vi "followUpDevice.vi"(8 "error in (no error)":errorcluster, 9 "S/N":string, 10 "Device Type":T1=enum."k4b2", 11 "reference in":refnum<class "Project Panels.lvclass">) -> (0 "error out":errorcluster, 3 "reference out":refnum<class "Project Panels.lvclass">)   [LabVIEW 2016, in "Project Panels.lvclass"]
uses:
  Project Panels.lvclass
  SYS/Devices Controller_llb/deviceType.ctl
  SYS/Devices Controller_llb/Devices Controller.lvclass
  SYS/File Controller_llb/File Controller.lvclass
  SYS/Notification Controller_class/Notification Controller.lvclass
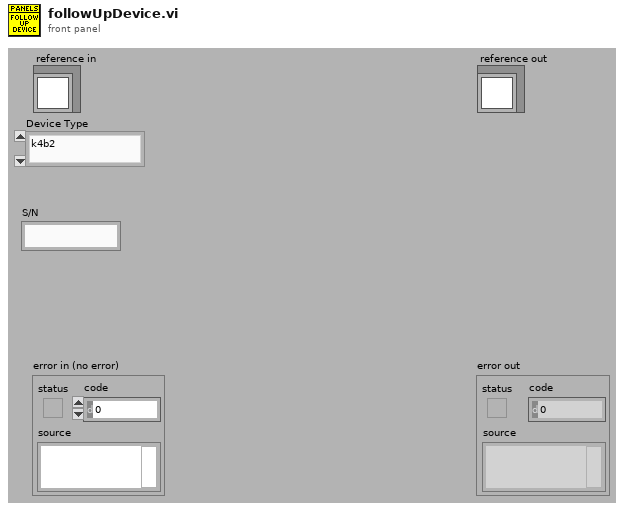
[diagram p1: front panel]
types:
  T1 = typedef "Devices Controller.lvclass/deviceType.ctl" = enum16{"k5", "k4b2", "fitmate", "cpet", "rmr", "bodyBoxPft", "bp", "pp"}
  T2 = typedef "Project Panels.lvclass/ObjectAttributesRef.ctl" = refnum<data-value>
  T3 = typedef "Project Panels.lvclass/ObjectAttributes.ctl" = cluster{"MyAttribute":dbl, "device_controller_ref":refnum<class "Devices Controller.lvclass">, "file_controller_ref":refnum<class "File Controller.lvclass">, "item_controller_ref":refnum<class "Items Controller.lvclass">, "item_tables":cluster{"checkIN":string[][], "checkOUT":string[][], "storage":string[][]}, "quickbook_table":cluster{"notes":string[][]}, "notification_controller_ref":refnum<class "Notification Controller.lvclass">, "partstracking_controller_ref":refnum<class "PartsTracking Controller.lvclass">, "product_tables":cluster{"k4b2":string[][], "fitmate":string[][], "RMR":string[][], "CPET":string[][], "BP":string[][], "PP":string[][], "k5":string[][], "bb-pft":string[][]}, "rowsColour":u32[], "low_resolution?":bool, "run_python?":bool}
  T4 = cluster{"deviceType":T1, "S/N":string, "SW":string, "Description":string, "Account":string, "System's Location":string, "End User":string, "Email":string, "City":string, "LastChange":string, "Service By":string, "Exp Date":string, "FollowUp Sent":string, "FollowUp Accepted":string, "Note":string}
  T5 = cluster{"filePaths":path[], "outlookTemplatePaths":path[], "attachmentTemplatePaths":path[]}
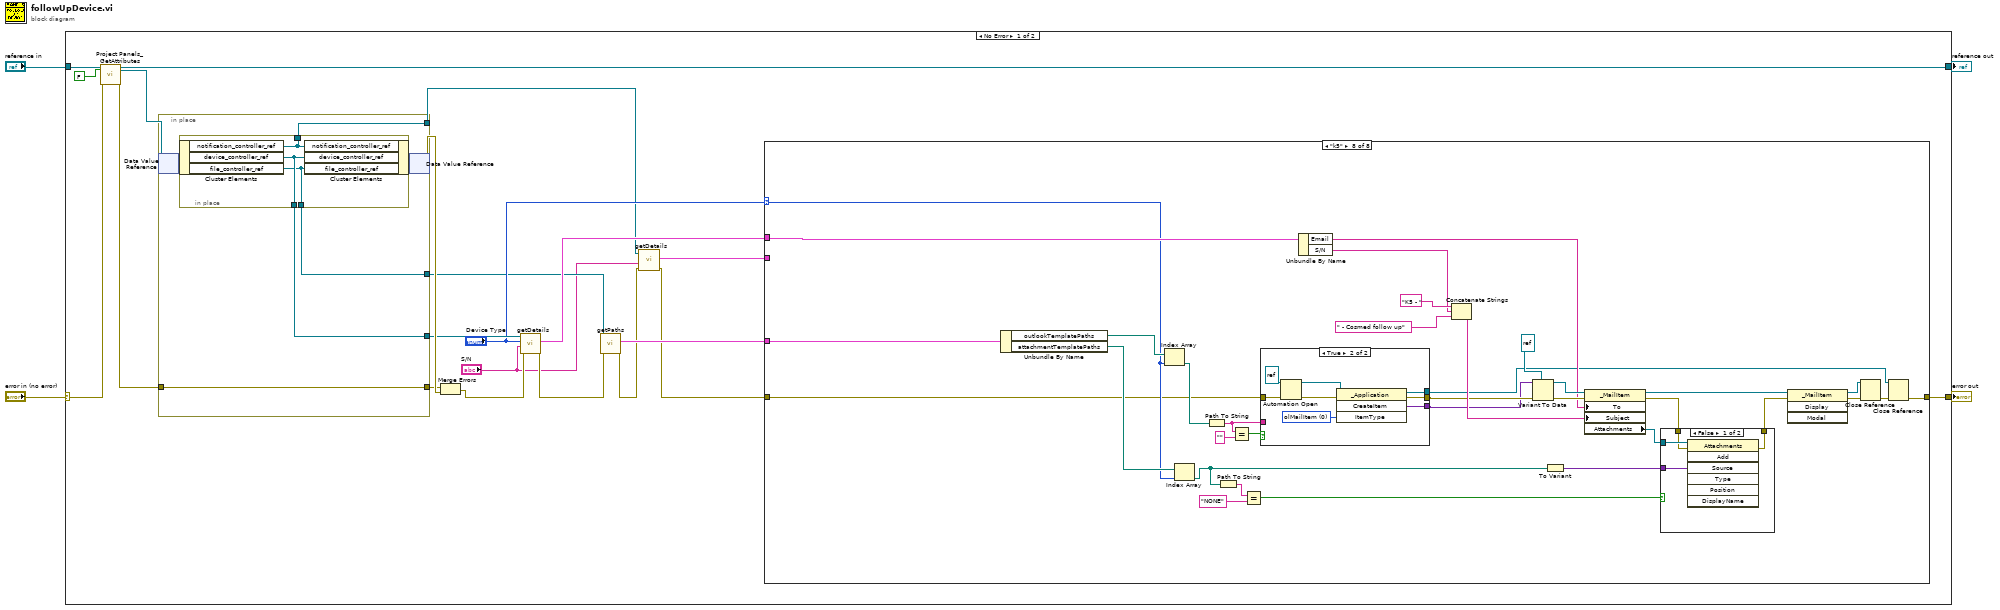
[diagram p0: block diagram]
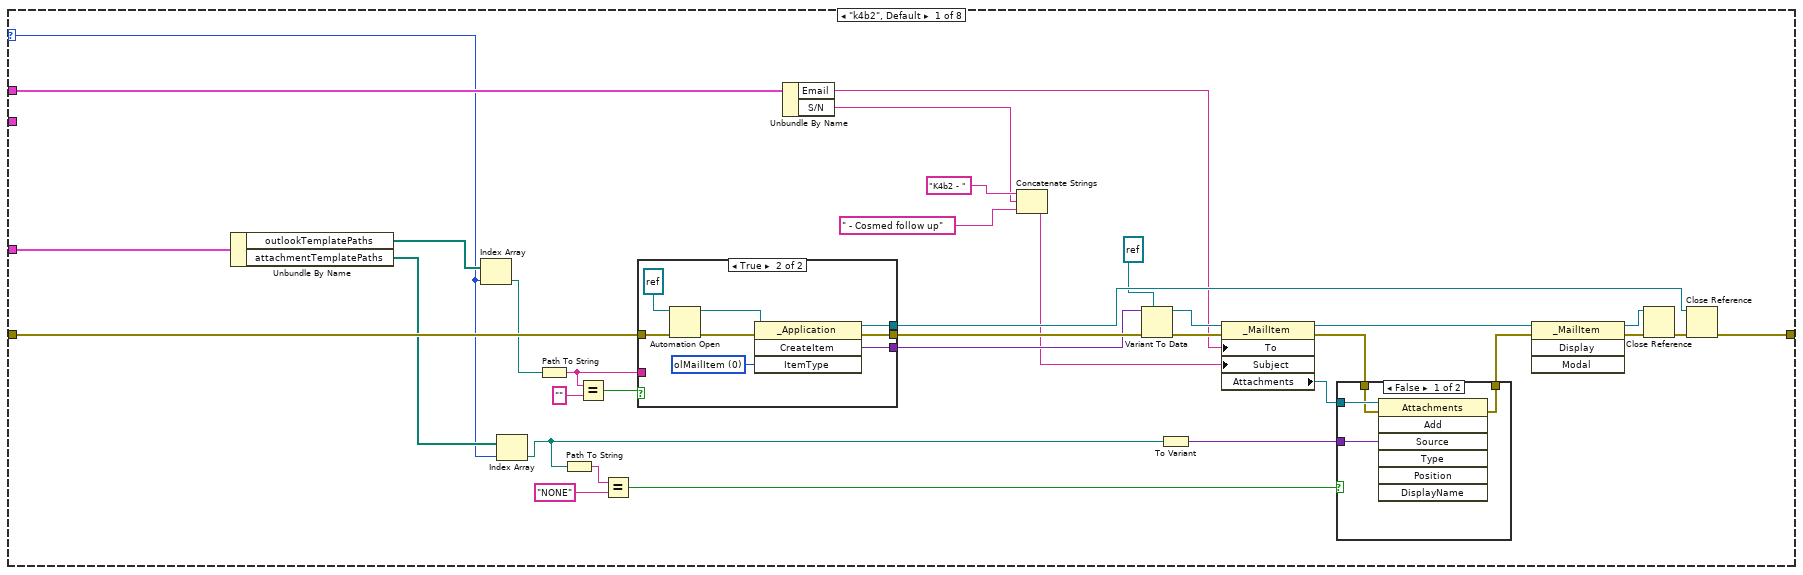
[diagram p2: hidden frame]
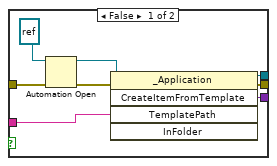
[diagram p3: hidden frame]
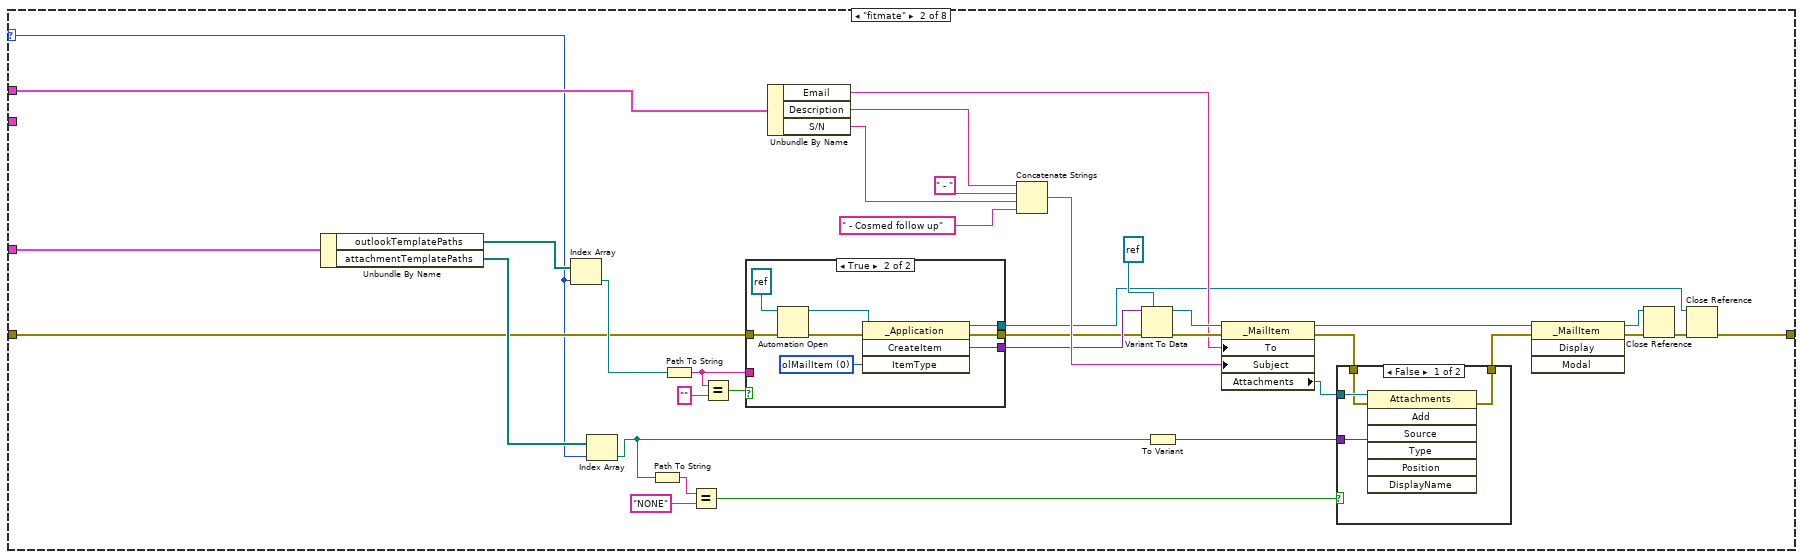
[diagram p5: hidden frame]
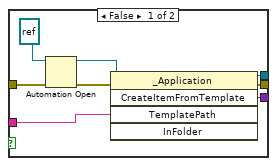
[diagram p6: hidden frame]
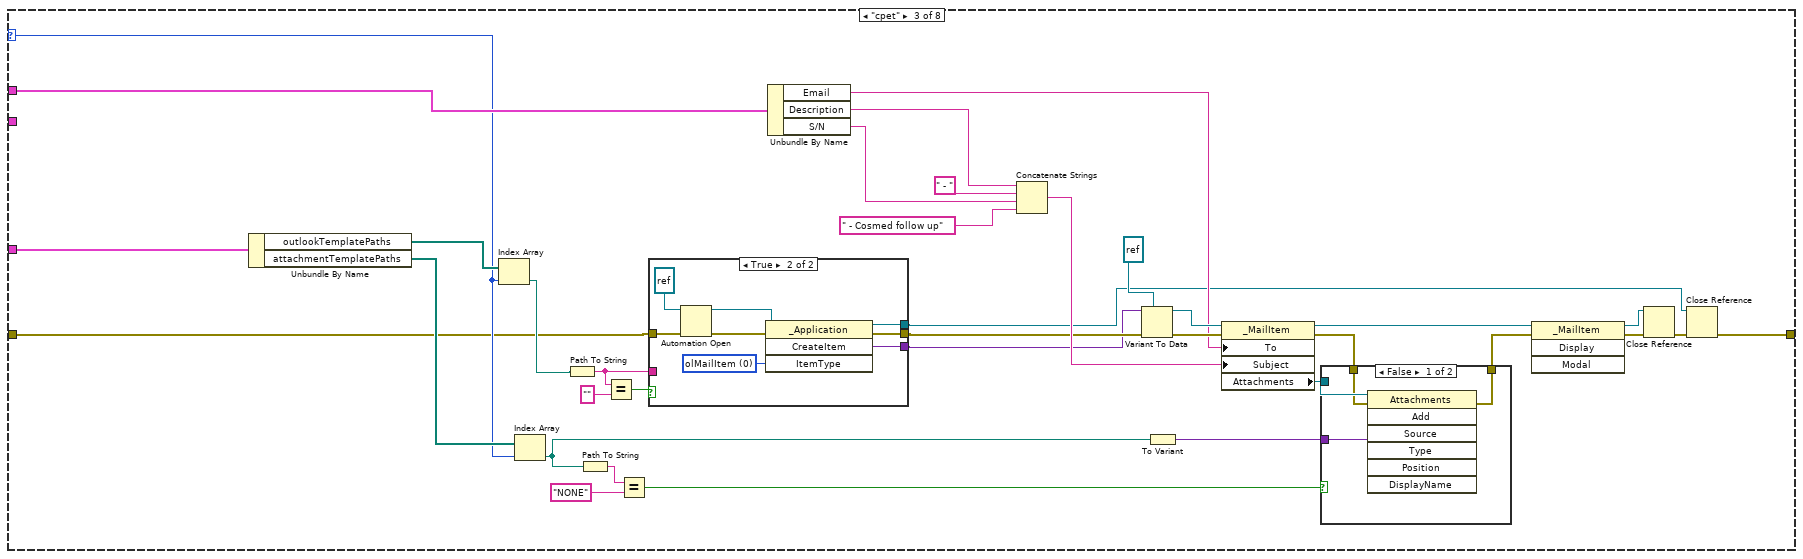
[diagram p8: hidden frame]
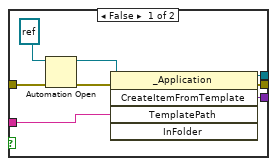
[diagram p9: hidden frame]
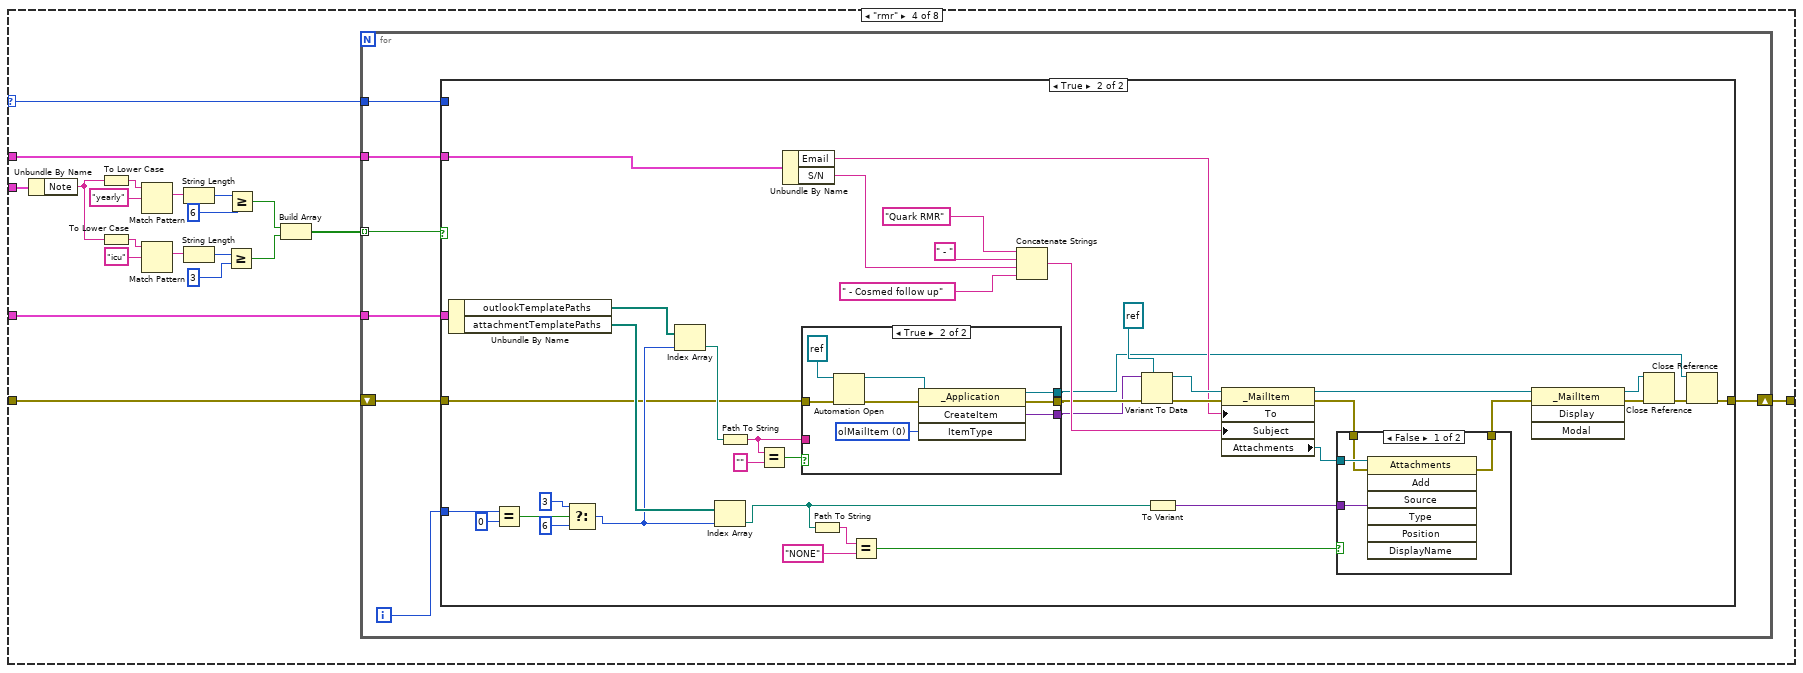
[diagram p11: hidden frame]
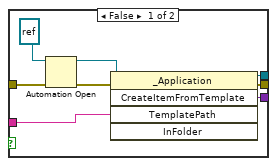
[diagram p13: hidden frame]
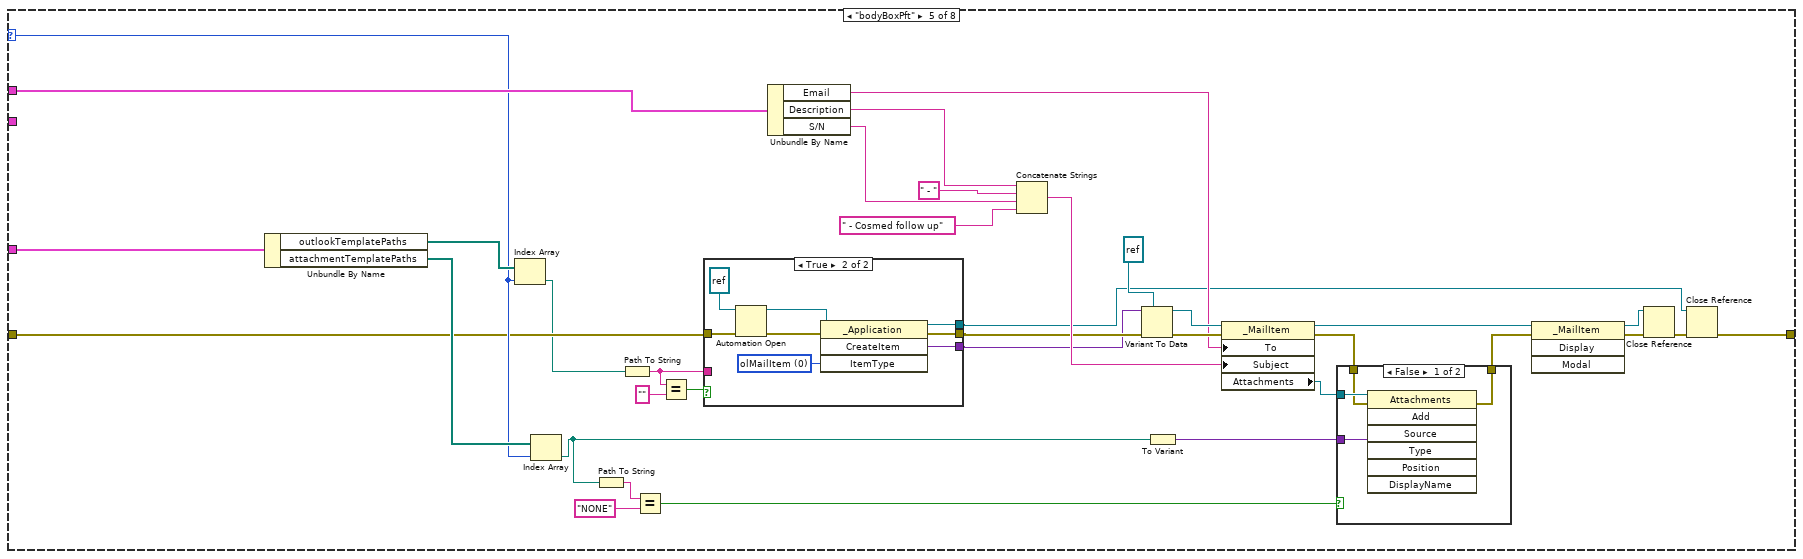
[diagram p15: hidden frame]
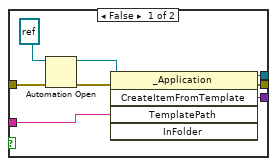
[diagram p16: hidden frame]
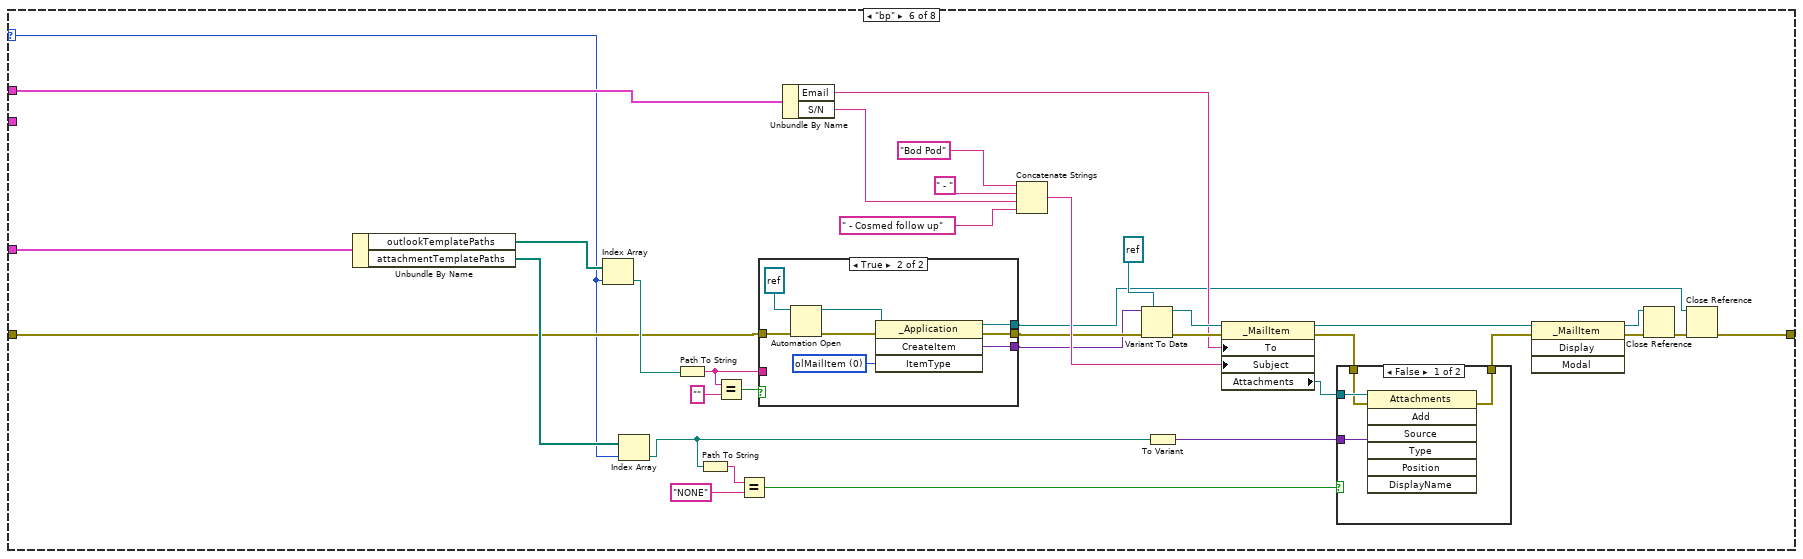
[diagram p18: hidden frame]
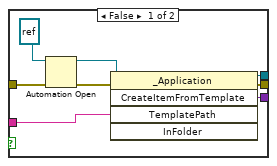
[diagram p19: hidden frame]
diagram:
  n1 = case shown="No Error" "error in (no error)" {
    selector: "error in (no error)" -> [w21 w514]
    tunnel: [w17 w514] -> w3
    tunnel: [w19 w513] -> w1
    tunnel: "reference in" -> [w23 w513]
    frame No Error {
      n2 = call "Project Panels_GetAttributes.vi"("reference in"=w23, "return data? (T)"=FALSE, "error in (no error)"=w21) -> ("reference out"=w19:refnum<class "Project Panels.lvclass">, "attributes ref"=w18:T2, "error out"=w20:errorcluster)  [unwired: 13 in, 1 out]
      n3 = in-place {
        in-place-border: w20 -> [w507]
        in-place-border: [w507] -> w24
        in-place-border: [w506] -> w15
        in-place-border: [w505] -> w12
        in-place-border: [w504] -> w5
        n4 = in-place-dvr #1(w18) -> (w508:T3)  [unwired: 1 out]
        n5 = in-place {
          in-place-border: [w512] -> w506
          in-place-border: [w511] -> w505
          in-place-border: [w510] -> w504
          n6 = in-place-cluster #2(w508) -> ("notification_controller_ref"=w510:refnum<class "Notification Controller.lvclass">, "device_controller_ref"=w512:refnum<class "Devices Controller.lvclass">, "file_controller_ref"=w511:refnum<class "File Controller.lvclass">)
          n7 = in-place-cluster #2("notification_controller_ref"=w510, "device_controller_ref"=w512, "file_controller_ref"=w511) -> (w509:T3)
        }
        n8 = in-place-dvr #1(w509) -> (w25:errorcluster)  [unwired: 1 out]
      }
      n9 = Merge Errors(w24, w25) -> (w16:errorcluster)
      n10 = call "getDetails.vi"("error in (no error)"=w16, "S/N"="S/N", "Device Type"="Device Type", "reference in"=w15) -> ("error out"=w11:errorcluster, "details"=w13:T4)  [unwired: 5 in, 1 out]
      n11 = call "getPaths.vi"("error in (no error)"=w11, "reference in"=w12) -> ("error out"=w8:errorcluster, "paths"=w10:T5)  [unwired: 7 in, 1 out]
      n12 = call "getDetails.vi"("error in (no error)"=w8, "S/N"="S/N", "reference in"=w5) -> ("error out"=w7:errorcluster, "details"=w9:T4)  [unwired: 6 in, 1 out]
      n13 = case shown="\"k5\"" "Device Type" {
        selector: "Device Type" -> [w29 w81 w145 w209 w291 w338 w402 w457]
        tunnel: [w49 w108 w164 w212 w309 w365 w403 w458] -> w17
        tunnel: w7 -> [w48 w85 w140 w211 w287 w342 w397 w452]
        tunnel: w13 -> [w47 w107 w163 w207 w308 w364 w404 w459]
        tunnel: w10 -> [w37 w94 w150 w210 w296 w352 w405 w460]
        tunnel: w9 -> [_ _ _ w208 _ _ _ _]
        frame "k4b2", Default {
          n14 = Unbundle By Name(w37) -> ("outlookTemplatePaths"=w36:path[], "attachmentTemplatePaths"=w35:path[])
          n15 = Index Array(array=w36, index=w29) -> (element=w34:path)
          n16 = Index Array(array=w35, index=w29) -> (element=w33:path)
          n17 = Path To String(path=w34) -> (string=w28:string)
          n18 = Path To String(path=w33) -> (string=w32:string)
          n19 = Equal?(x=w28, y="") -> (x = y?=w26:bool)
          n20 = Equal?(x=w32, y="NONE") -> (x = y?=w30:bool)
          n21 = case shown="True" w26 {
            tunnel: [w66 w69] -> w56
            tunnel: [w65 w70] -> w55
            tunnel: [w63 w71] -> w54
            tunnel: w48 -> [w61 w72]
            tunnel: w28 -> [w60 _]
            frame False {
              n22 = Automation Open(error in (no error)=w61, Automation Refnum=refnum<k7> refnum ("Outlook._Application")) -> (Automation Refnum=w67:refnum<k7>, error out=w62:errorcluster)  [unwired: 2 in]
              n23 = invoke class="_Application" method="CreateItemFromTemplate"(reference=w67, error in=w62, "TemplatePath"=w60) -> (reference out=w66:refnum<k7>, error out=w65:errorcluster, "CreateItemFromTemplate"=w63:variant)  [unwired: 2 in, 2 out]
            }
            frame True {
              w68 = 0 items=["olMailItem"=0, "olAppointmentItem"=1, "olContactItem"=2, "olTaskItem"=3, "olJournalItem"=4, "olNoteItem"=5, "olPostItem"=6, "olDistributionListItem"=7, "olMobileItemSMS"=11, "olMobileItemMMS"=12] ("ItemType")
              n24 = Automation Open(error in (no error)=w72, Automation Refnum=refnum<k7> refnum ("Outlook._Application")) -> (Automation Refnum=w75:refnum<k7>, error out=w74:errorcluster)  [unwired: 2 in]
              n25 = invoke class="_Application" method="CreateItem"(reference=w75, error in=w74, "ItemType"=w68) -> (reference out=w69:refnum<k7>, error out=w70:errorcluster, "CreateItem"=w71:variant)  [unwired: 1 in, 1 out]
            }
          }
          n26 = Unbundle By Name(w47) -> ("Email"=w46:string, "S/N"=w44:string)
          n27 = Concatenate Strings("K4b2 - " ("string"), w44, " - Cosmed follow up" ("string")) -> (w42:string)
          n28 = Variant To Data(error in=w55, type=refnum<k7> refnum ("Outlook._MailItem"), Variant=w54) -> (data=w57:refnum<k7>, error out=w50:errorcluster)
          n29 = To Variant(anything=w33) -> (Variant=w38:variant)
          n30 = property class="_MailItem"(reference=w57, error in=w50, "To"=w46, "Subject"=w42) -> (reference out=w58:refnum<k7>, error out=w40:errorcluster, "Attachments"=w41:refnum<k7>)
          n31 = case shown="False" w30 {
            tunnel: w41 -> [w79 _]
            tunnel: w40 -> [w78 w80]
            tunnel: [w77 w80] -> w39
            tunnel: w38 -> [w76 _]
            frame False {
              n32 = invoke class="Attachments" method="Add"(reference=w79, error in=w78, "Source"=w76) -> (error out=w77:errorcluster)  [unwired: 4 in, 6 out]
            }
            frame True {
            }
          }
          n33 = invoke class="_MailItem" method="Display"(reference=w58, error in=w39) -> (reference out=w52:refnum<k7>, error out=w51:errorcluster)  [unwired: 2 in, 2 out]
          n34 = Close Reference(reference=w52, error in (no error)=w51) -> (error out=w59:errorcluster)
          n35 = Close Reference(reference=w56, error in (no error)=w59) -> (error out=w49:errorcluster)
        }
        frame "fitmate" {
          n36 = Unbundle By Name(w94) -> ("outlookTemplatePaths"=w96:path[], "attachmentTemplatePaths"=w95:path[])
          n37 = Index Array(array=w96, index=w81) -> (element=w86:path)
          n38 = Index Array(array=w95, index=w81) -> (element=w91:path)
          n39 = Path To String(path=w91) -> (string=w93:string)
          n40 = Path To String(path=w86) -> (string=w89:string)
          n41 = Equal?(x=w93, y="NONE") -> (x = y?=w90:bool)
          n42 = Equal?(x=w89, y="") -> (x = y?=w87:bool)
          n43 = case shown="True" w87 {
            tunnel: [w122 w125] -> w84
            tunnel: [w121 w126] -> w82
            tunnel: [w119 w127] -> w83
            tunnel: w85 -> [w117 w128]
            tunnel: w89 -> [w116 _]
            frame False {
              n44 = Automation Open(error in (no error)=w117, Automation Refnum=refnum<k7> refnum ("Outlook._Application")) -> (Automation Refnum=w123:refnum<k7>, error out=w118:errorcluster)  [unwired: 2 in]
              n45 = invoke class="_Application" method="CreateItemFromTemplate"(reference=w123, error in=w118, "TemplatePath"=w116) -> (reference out=w122:refnum<k7>, error out=w121:errorcluster, "CreateItemFromTemplate"=w119:variant)  [unwired: 2 in, 2 out]
            }
            frame True {
              w124 = 0 items=["olMailItem"=0, "olAppointmentItem"=1, "olContactItem"=2, "olTaskItem"=3, "olJournalItem"=4, "olNoteItem"=5, "olPostItem"=6, "olDistributionListItem"=7, "olMobileItemSMS"=11, "olMobileItemMMS"=12] ("ItemType")
              n46 = Automation Open(error in (no error)=w128, Automation Refnum=refnum<k7> refnum ("Outlook._Application")) -> (Automation Refnum=w131:refnum<k7>, error out=w130:errorcluster)  [unwired: 2 in]
              n47 = invoke class="_Application" method="CreateItem"(reference=w131, error in=w130, "ItemType"=w124) -> (reference out=w125:refnum<k7>, error out=w126:errorcluster, "CreateItem"=w127:variant)  [unwired: 1 in, 1 out]
            }
          }
          n48 = Unbundle By Name(w107) -> ("Email"=w106:string, "Description"=w103:string, "S/N"=w101:string)
          n49 = Concatenate Strings(w103, " - " ("string"), w101, " - Cosmed follow up" ("string")) -> (w104:string)
          n50 = Variant To Data(error in=w82, type=refnum<k7> refnum ("Outlook._MailItem"), Variant=w83) -> (data=w113:refnum<k7>, error out=w109:errorcluster)
          n51 = To Variant(anything=w91) -> (Variant=w97:variant)
          n52 = property class="_MailItem"(reference=w113, error in=w109, "To"=w106, "Subject"=w104) -> (reference out=w114:refnum<k7>, error out=w99:errorcluster, "Attachments"=w100:refnum<k7>)
          n53 = case shown="False" w90 {
            tunnel: w100 -> [w135 _]
            tunnel: w99 -> [w134 w136]
            tunnel: [w133 w136] -> w98
            tunnel: w97 -> [w132 _]
            frame False {
              n54 = invoke class="Attachments" method="Add"(reference=w135, error in=w134, "Source"=w132) -> (error out=w133:errorcluster)  [unwired: 4 in, 6 out]
            }
            frame True {
            }
          }
          n55 = invoke class="_MailItem" method="Display"(reference=w114, error in=w98) -> (reference out=w111:refnum<k7>, error out=w110:errorcluster)  [unwired: 2 in, 2 out]
          n56 = Close Reference(reference=w111, error in (no error)=w110) -> (error out=w115:errorcluster)
          n57 = Close Reference(reference=w84, error in (no error)=w115) -> (error out=w108:errorcluster)
        }
        frame "cpet" {
          n58 = Unbundle By Name(w150) -> ("outlookTemplatePaths"=w152:path[], "attachmentTemplatePaths"=w151:path[])
          n59 = Index Array(array=w152, index=w145) -> (element=w141:path)
          n60 = Index Array(array=w151, index=w145) -> (element=w147:path)
          n61 = Path To String(path=w141) -> (string=w144:string)
          n62 = Path To String(path=w147) -> (string=w149:string)
          n63 = Equal?(x=w144, y="") -> (x = y?=w142:bool)
          n64 = Equal?(x=w149, y="NONE") -> (x = y?=w146:bool)
          n65 = case shown="True" w142 {
            tunnel: [w178 w181] -> w139
            tunnel: [w177 w182] -> w138
            tunnel: [w175 w183] -> w137
            tunnel: w140 -> [w173 w184]
            tunnel: w144 -> [w172 _]
            frame False {
              n66 = Automation Open(error in (no error)=w173, Automation Refnum=refnum<k7> refnum ("Outlook._Application")) -> (Automation Refnum=w179:refnum<k7>, error out=w174:errorcluster)  [unwired: 2 in]
              n67 = invoke class="_Application" method="CreateItemFromTemplate"(reference=w179, error in=w174, "TemplatePath"=w172) -> (reference out=w178:refnum<k7>, error out=w177:errorcluster, "CreateItemFromTemplate"=w175:variant)  [unwired: 2 in, 2 out]
            }
            frame True {
              w180 = 0 items=["olMailItem"=0, "olAppointmentItem"=1, "olContactItem"=2, "olTaskItem"=3, "olJournalItem"=4, "olNoteItem"=5, "olPostItem"=6, "olDistributionListItem"=7, "olMobileItemSMS"=11, "olMobileItemMMS"=12] ("ItemType")
              n68 = Automation Open(error in (no error)=w184, Automation Refnum=refnum<k7> refnum ("Outlook._Application")) -> (Automation Refnum=w187:refnum<k7>, error out=w186:errorcluster)  [unwired: 2 in]
              n69 = invoke class="_Application" method="CreateItem"(reference=w187, error in=w186, "ItemType"=w180) -> (reference out=w181:refnum<k7>, error out=w182:errorcluster, "CreateItem"=w183:variant)  [unwired: 1 in, 1 out]
            }
          }
          n70 = Unbundle By Name(w163) -> ("Email"=w162:string, "Description"=w159:string, "S/N"=w157:string)
          n71 = Concatenate Strings(w159, " - " ("string"), w157, " - Cosmed follow up" ("string")) -> (w160:string)
          n72 = Variant To Data(error in=w138, type=refnum<k7> refnum ("Outlook._MailItem"), Variant=w137) -> (data=w169:refnum<k7>, error out=w165:errorcluster)
          n73 = To Variant(anything=w147) -> (Variant=w153:variant)
          n74 = property class="_MailItem"(reference=w169, error in=w165, "To"=w162, "Subject"=w160) -> (reference out=w170:refnum<k7>, error out=w155:errorcluster, "Attachments"=w156:refnum<k7>)
          n75 = case shown="False" w146 {
            tunnel: w156 -> [w191 _]
            tunnel: w155 -> [w190 w192]
            tunnel: [w189 w192] -> w154
            tunnel: w153 -> [w188 _]
            frame False {
              n76 = invoke class="Attachments" method="Add"(reference=w191, error in=w190, "Source"=w188) -> (error out=w189:errorcluster)  [unwired: 4 in, 6 out]
            }
            frame True {
            }
          }
          n77 = invoke class="_MailItem" method="Display"(reference=w170, error in=w154) -> (reference out=w167:refnum<k7>, error out=w166:errorcluster)  [unwired: 2 in, 2 out]
          n78 = Close Reference(reference=w167, error in (no error)=w166) -> (error out=w171:errorcluster)
          n79 = Close Reference(reference=w139, error in (no error)=w171) -> (error out=w164:errorcluster)
        }
        frame "rmr" {
          n80 = Unbundle By Name(w208) -> ("Note"=w200:string)
          n81 = To Lower Case(string=w200) -> (all lower case string=w201:string)
          n82 = To Lower Case(string=w200) -> (all lower case string=w206:string)
          n83 = Match Pattern(string=w201, regular expression="yearly") -> (match substring=w203:string)  [unwired: 1 in, 3 out]
          n84 = Match Pattern(string=w206, regular expression="icu") -> (match substring=w204:string)  [unwired: 1 in, 3 out]
          n85 = String Length(string=w203) -> (length=w199:i32)
          n86 = String Length(string=w204) -> (length=w198:i32)
          n87 = Greater Or Equal?(x=w198, y=3) -> (x >= y?=w195:bool)
          n88 = Greater Or Equal?(x=w199, y=6) -> (x >= y?=w194:bool)
          n89 = Build Array(w194, w195) -> (w193:bool[])
          n90 = for {
            tunnel: w210 -> [w217]
            tunnel: w209 -> [w216]
            tunnel: w207 -> [w215]
            shift-right: [w219] -> w212
            shift-left: w211 -> [w218]
            tunnel: w193 -> [w214] mode=indexing
            i -> [w213]
            n91 = case shown="True" w214 {
              tunnel: [w220 w253] -> w219
              tunnel: w218 -> [w220 w224]
              tunnel: w217 -> [_ w241]
              tunnel: w216 -> [_ _]
              tunnel: w215 -> [_ w240]
              tunnel: w213 -> [_ w239]
              frame False {
              }
              frame True {
                n92 = Unbundle By Name(w241) -> ("outlookTemplatePaths"=w243:path[], "attachmentTemplatePaths"=w242:path[])
                n93 = Equal?(x=w239, y=0) -> (x = y?=w237:bool)
                n94 = Select(t=3 ("y"), s=w237, f=6) -> (s? t:f=w234:i32)
                n95 = Index Array(array=w243, index=w234) -> (element=w225:path)
                n96 = Index Array(array=w242, index=w234) -> (element=w230:path)
                n97 = Path To String(path=w225) -> (string=w228:string)
                n98 = Equal?(x=w228, y="") -> (x = y?=w226:bool)
                n99 = Unbundle By Name(w240) -> ("Email"=w252:string, "S/N"=w248:string)
                n100 = case shown="True" w226 {
                  tunnel: [w267 w270] -> w223
                  tunnel: [w266 w271] -> w222
                  tunnel: [w264 w272] -> w221
                  tunnel: w224 -> [w262 w273]
                  tunnel: w228 -> [w261 _]
                  frame False {
                    n101 = Automation Open(error in (no error)=w262, Automation Refnum=refnum<k7> refnum ("Outlook._Application")) -> (Automation Refnum=w268:refnum<k7>, error out=w263:errorcluster)  [unwired: 2 in]
                    n102 = invoke class="_Application" method="CreateItemFromTemplate"(reference=w268, error in=w263, "TemplatePath"=w261) -> (reference out=w267:refnum<k7>, error out=w266:errorcluster, "CreateItemFromTemplate"=w264:variant)  [unwired: 2 in, 2 out]
                  }
                  frame True {
                    w269 = 0 items=["olMailItem"=0, "olAppointmentItem"=1, "olContactItem"=2, "olTaskItem"=3, "olJournalItem"=4, "olNoteItem"=5, "olPostItem"=6, "olDistributionListItem"=7, "olMobileItemSMS"=11, "olMobileItemMMS"=12] ("ItemType")
                    n103 = Automation Open(error in (no error)=w273, Automation Refnum=refnum<k7> refnum ("Outlook._Application")) -> (Automation Refnum=w276:refnum<k7>, error out=w275:errorcluster)  [unwired: 2 in]
                    n104 = invoke class="_Application" method="CreateItem"(reference=w276, error in=w275, "ItemType"=w269) -> (reference out=w270:refnum<k7>, error out=w271:errorcluster, "CreateItem"=w272:variant)  [unwired: 1 in, 1 out]
                  }
                }
                n105 = Path To String(path=w230) -> (string=w232:string)
                n106 = Equal?(x=w232, y="NONE") -> (x = y?=w229:bool)
                n107 = Concatenate Strings("Quark RMR" ("string"), " - " ("string"), w248, " - Cosmed follow up" ("string")) -> (w250:string)
                n108 = Variant To Data(error in=w222, type=refnum<k7> refnum ("Outlook._MailItem"), Variant=w221) -> (data=w258:refnum<k7>, error out=w254:errorcluster)
                n109 = To Variant(anything=w230) -> (Variant=w244:variant)
                n110 = property class="_MailItem"(reference=w258, error in=w254, "To"=w252, "Subject"=w250) -> (reference out=w259:refnum<k7>, error out=w246:errorcluster, "Attachments"=w247:refnum<k7>)
                n111 = case shown="False" w229 {
                  tunnel: w247 -> [w280 _]
                  tunnel: w246 -> [w279 w281]
                  tunnel: [w278 w281] -> w245
                  tunnel: w244 -> [w277 _]
                  frame False {
                    n112 = invoke class="Attachments" method="Add"(reference=w280, error in=w279, "Source"=w277) -> (error out=w278:errorcluster)  [unwired: 4 in, 6 out]
                  }
                  frame True {
                  }
                }
                n113 = invoke class="_MailItem" method="Display"(reference=w259, error in=w245) -> (reference out=w256:refnum<k7>, error out=w255:errorcluster)  [unwired: 2 in, 2 out]
                n114 = Close Reference(reference=w256, error in (no error)=w255) -> (error out=w260:errorcluster)
                n115 = Close Reference(reference=w223, error in (no error)=w260) -> (error out=w253:errorcluster)
              }
            }
          }
        }
        frame "bodyBoxPft" {
          n116 = Unbundle By Name(w296) -> ("outlookTemplatePaths"=w298:path[], "attachmentTemplatePaths"=w297:path[])
          n117 = Index Array(array=w298, index=w291) -> (element=w286:path)
          n118 = Index Array(array=w297, index=w291) -> (element=w293:path)
          n119 = Path To String(path=w293) -> (string=w295:string)
          n120 = Path To String(path=w286) -> (string=w290:string)
          n121 = Equal?(x=w295, y="NONE") -> (x = y?=w292:bool)
          n122 = Equal?(x=w290, y="") -> (x = y?=w288:bool)
          n123 = case shown="True" w288 {
            tunnel: [w323 w326] -> w285
            tunnel: [w322 w327] -> w284
            tunnel: [w320 w328] -> w283
            tunnel: w287 -> [w318 w329]
            tunnel: w290 -> [w317 _]
            frame False {
              n124 = Automation Open(error in (no error)=w318, Automation Refnum=refnum<k7> refnum ("Outlook._Application")) -> (Automation Refnum=w324:refnum<k7>, error out=w319:errorcluster)  [unwired: 2 in]
              n125 = invoke class="_Application" method="CreateItemFromTemplate"(reference=w324, error in=w319, "TemplatePath"=w317) -> (reference out=w323:refnum<k7>, error out=w322:errorcluster, "CreateItemFromTemplate"=w320:variant)  [unwired: 2 in, 2 out]
            }
            frame True {
              w325 = 0 items=["olMailItem"=0, "olAppointmentItem"=1, "olContactItem"=2, "olTaskItem"=3, "olJournalItem"=4, "olNoteItem"=5, "olPostItem"=6, "olDistributionListItem"=7, "olMobileItemSMS"=11, "olMobileItemMMS"=12] ("ItemType")
              n126 = Automation Open(error in (no error)=w329, Automation Refnum=refnum<k7> refnum ("Outlook._Application")) -> (Automation Refnum=w332:refnum<k7>, error out=w331:errorcluster)  [unwired: 2 in]
              n127 = invoke class="_Application" method="CreateItem"(reference=w332, error in=w331, "ItemType"=w325) -> (reference out=w326:refnum<k7>, error out=w327:errorcluster, "CreateItem"=w328:variant)  [unwired: 1 in, 1 out]
            }
          }
          n128 = Unbundle By Name(w308) -> ("Email"=w307:string, "Description"=w282:string, "S/N"=w303:string)
          n129 = Concatenate Strings(w282, " - " ("string"), w303, " - Cosmed follow up" ("string")) -> (w305:string)
          n130 = Variant To Data(error in=w284, type=refnum<k7> refnum ("Outlook._MailItem"), Variant=w283) -> (data=w314:refnum<k7>, error out=w310:errorcluster)
          n131 = To Variant(anything=w293) -> (Variant=w299:variant)
          n132 = property class="_MailItem"(reference=w314, error in=w310, "To"=w307, "Subject"=w305) -> (reference out=w315:refnum<k7>, error out=w301:errorcluster, "Attachments"=w302:refnum<k7>)
          n133 = case shown="False" w292 {
            tunnel: w302 -> [w336 _]
            tunnel: w301 -> [w335 w337]
            tunnel: [w334 w337] -> w300
            tunnel: w299 -> [w333 _]
            frame False {
              n134 = invoke class="Attachments" method="Add"(reference=w336, error in=w335, "Source"=w333) -> (error out=w334:errorcluster)  [unwired: 4 in, 6 out]
            }
            frame True {
            }
          }
          n135 = invoke class="_MailItem" method="Display"(reference=w315, error in=w300) -> (reference out=w312:refnum<k7>, error out=w311:errorcluster)  [unwired: 2 in, 2 out]
          n136 = Close Reference(reference=w312, error in (no error)=w311) -> (error out=w316:errorcluster)
          n137 = Close Reference(reference=w285, error in (no error)=w316) -> (error out=w309:errorcluster)
        }
        frame "bp" {
          n138 = Unbundle By Name(w352) -> ("outlookTemplatePaths"=w354:path[], "attachmentTemplatePaths"=w353:path[])
          n139 = Index Array(array=w354, index=w338) -> (element=w343:path)
          n140 = Index Array(array=w353, index=w338) -> (element=w349:path)
          n141 = Path To String(path=w343) -> (string=w346:string)
          n142 = Path To String(path=w349) -> (string=w351:string)
          n143 = Equal?(x=w346, y="") -> (x = y?=w344:bool)
          n144 = Equal?(x=w351, y="NONE") -> (x = y?=w348:bool)
          n145 = case shown="True" w344 {
            tunnel: [w379 w382] -> w341
            tunnel: [w378 w383] -> w340
            tunnel: [w376 w384] -> w339
            tunnel: w342 -> [w374 w385]
            tunnel: w346 -> [w373 _]
            frame False {
              n146 = Automation Open(error in (no error)=w374, Automation Refnum=refnum<k7> refnum ("Outlook._Application")) -> (Automation Refnum=w380:refnum<k7>, error out=w375:errorcluster)  [unwired: 2 in]
              n147 = invoke class="_Application" method="CreateItemFromTemplate"(reference=w380, error in=w375, "TemplatePath"=w373) -> (reference out=w379:refnum<k7>, error out=w378:errorcluster, "CreateItemFromTemplate"=w376:variant)  [unwired: 2 in, 2 out]
            }
            frame True {
              w381 = 0 items=["olMailItem"=0, "olAppointmentItem"=1, "olContactItem"=2, "olTaskItem"=3, "olJournalItem"=4, "olNoteItem"=5, "olPostItem"=6, "olDistributionListItem"=7, "olMobileItemSMS"=11, "olMobileItemMMS"=12] ("ItemType")
              n148 = Automation Open(error in (no error)=w385, Automation Refnum=refnum<k7> refnum ("Outlook._Application")) -> (Automation Refnum=w388:refnum<k7>, error out=w387:errorcluster)  [unwired: 2 in]
              n149 = invoke class="_Application" method="CreateItem"(reference=w388, error in=w387, "ItemType"=w381) -> (reference out=w382:refnum<k7>, error out=w383:errorcluster, "CreateItem"=w384:variant)  [unwired: 1 in, 1 out]
            }
          }
          n150 = Unbundle By Name(w364) -> ("Email"=w363:string, "S/N"=w359:string)
          n151 = Concatenate Strings("Bod Pod" ("string"), " - " ("string"), w359, " - Cosmed follow up" ("string")) -> (w361:string)
          n152 = Variant To Data(error in=w340, type=refnum<k7> refnum ("Outlook._MailItem"), Variant=w339) -> (data=w370:refnum<k7>, error out=w366:errorcluster)
          n153 = To Variant(anything=w349) -> (Variant=w355:variant)
          n154 = property class="_MailItem"(reference=w370, error in=w366, "To"=w363, "Subject"=w361) -> (reference out=w371:refnum<k7>, error out=w357:errorcluster, "Attachments"=w358:refnum<k7>)
          n155 = case shown="False" w348 {
            tunnel: w358 -> [w392 _]
            tunnel: w357 -> [w391 w393]
            tunnel: [w390 w393] -> w356
            tunnel: w355 -> [w389 _]
            frame False {
              n156 = invoke class="Attachments" method="Add"(reference=w392, error in=w391, "Source"=w389) -> (error out=w390:errorcluster)  [unwired: 4 in, 6 out]
            }
            frame True {
            }
          }
          n157 = invoke class="_MailItem" method="Display"(reference=w371, error in=w356) -> (reference out=w368:refnum<k7>, error out=w367:errorcluster)  [unwired: 2 in, 2 out]
          n158 = Close Reference(reference=w368, error in (no error)=w367) -> (error out=w372:errorcluster)
          n159 = Close Reference(reference=w341, error in (no error)=w372) -> (error out=w365:errorcluster)
        }
        frame "pp" {
          n160 = Unbundle By Name(w405) -> ("outlookTemplatePaths"=w411:path[], "attachmentTemplatePaths"=w410:path[])
          n161 = Index Array(array=w411, index=w402) -> (element=w398:path)
          n162 = Index Array(array=w410, index=w402) -> (element=w409:path)
          n163 = Path To String(path=w398) -> (string=w401:string)
          n164 = Path To String(path=w409) -> (string=w408:string)
          n165 = Equal?(x=w401, y="") -> (x = y?=w399:bool)
          n166 = Equal?(x=w408, y="NONE") -> (x = y?=w406:bool)
          n167 = case shown="True" w399 {
            tunnel: [w434 w437] -> w396
            tunnel: [w433 w438] -> w395
            tunnel: [w431 w439] -> w394
            tunnel: w397 -> [w429 w440]
            tunnel: w401 -> [w428 _]
            frame False {
              n168 = Automation Open(error in (no error)=w429, Automation Refnum=refnum<k7> refnum ("Outlook._Application")) -> (Automation Refnum=w435:refnum<k7>, error out=w430:errorcluster)  [unwired: 2 in]
              n169 = invoke class="_Application" method="CreateItemFromTemplate"(reference=w435, error in=w430, "TemplatePath"=w428) -> (reference out=w434:refnum<k7>, error out=w433:errorcluster, "CreateItemFromTemplate"=w431:variant)  [unwired: 2 in, 2 out]
            }
            frame True {
              w436 = 0 items=["olMailItem"=0, "olAppointmentItem"=1, "olContactItem"=2, "olTaskItem"=3, "olJournalItem"=4, "olNoteItem"=5, "olPostItem"=6, "olDistributionListItem"=7, "olMobileItemSMS"=11, "olMobileItemMMS"=12] ("ItemType")
              n170 = Automation Open(error in (no error)=w440, Automation Refnum=refnum<k7> refnum ("Outlook._Application")) -> (Automation Refnum=w443:refnum<k7>, error out=w442:errorcluster)  [unwired: 2 in]
              n171 = invoke class="_Application" method="CreateItem"(reference=w443, error in=w442, "ItemType"=w436) -> (reference out=w437:refnum<k7>, error out=w438:errorcluster, "CreateItem"=w439:variant)  [unwired: 1 in, 1 out]
            }
          }
          n172 = Unbundle By Name(w404) -> ("Email"=w420:string, "S/N"=w418:string)
          n173 = Concatenate Strings("Pea Pod - " ("string"), w418, " - Cosmed follow up" ("string")) -> (w416:string)
          n174 = Variant To Data(error in=w395, type=refnum<k7> refnum ("Outlook._MailItem"), Variant=w394) -> (data=w425:refnum<k7>, error out=w421:errorcluster)
          n175 = To Variant(anything=w409) -> (Variant=w412:variant)
          n176 = property class="_MailItem"(reference=w425, error in=w421, "To"=w420, "Subject"=w416) -> (reference out=w426:refnum<k7>, error out=w414:errorcluster, "Attachments"=w415:refnum<k7>)
          n177 = case shown="False" w406 {
            tunnel: w415 -> [w447 _]
            tunnel: w414 -> [w446 w448]
            tunnel: [w445 w448] -> w413
            tunnel: w412 -> [w444 _]
            frame False {
              n178 = invoke class="Attachments" method="Add"(reference=w447, error in=w446, "Source"=w444) -> (error out=w445:errorcluster)  [unwired: 4 in, 6 out]
            }
            frame True {
            }
          }
          n179 = invoke class="_MailItem" method="Display"(reference=w426, error in=w413) -> (reference out=w423:refnum<k7>, error out=w422:errorcluster)  [unwired: 2 in, 2 out]
          n180 = Close Reference(reference=w423, error in (no error)=w422) -> (error out=w427:errorcluster)
          n181 = Close Reference(reference=w396, error in (no error)=w427) -> (error out=w403:errorcluster)
        }
        frame "k5" {
          n182 = Unbundle By Name(w460) -> ("outlookTemplatePaths"=w466:path[], "attachmentTemplatePaths"=w465:path[])
          n183 = Index Array(array=w466, index=w457) -> (element=w453:path)
          n184 = Index Array(array=w465, index=w457) -> (element=w464:path)
          n185 = Path To String(path=w453) -> (string=w456:string)
          n186 = Path To String(path=w464) -> (string=w463:string)
          n187 = Equal?(x=w456, y="") -> (x = y?=w454:bool)
          n188 = Equal?(x=w463, y="NONE") -> (x = y?=w461:bool)
          n189 = case shown="True" w454 {
            tunnel: [w489 w492] -> w451
            tunnel: [w488 w493] -> w450
            tunnel: [w486 w494] -> w449
            tunnel: w452 -> [w484 w495]
            tunnel: w456 -> [w483 _]
            frame False {
              n190 = Automation Open(error in (no error)=w484, Automation Refnum=refnum<k7> refnum ("Outlook._Application")) -> (Automation Refnum=w490:refnum<k7>, error out=w485:errorcluster)  [unwired: 2 in]
              n191 = invoke class="_Application" method="CreateItemFromTemplate"(reference=w490, error in=w485, "TemplatePath"=w483) -> (reference out=w489:refnum<k7>, error out=w488:errorcluster, "CreateItemFromTemplate"=w486:variant)  [unwired: 2 in, 2 out]
            }
            frame True {
              w491 = 0 items=["olMailItem"=0, "olAppointmentItem"=1, "olContactItem"=2, "olTaskItem"=3, "olJournalItem"=4, "olNoteItem"=5, "olPostItem"=6, "olDistributionListItem"=7, "olMobileItemSMS"=11, "olMobileItemMMS"=12] ("ItemType")
              n192 = Automation Open(error in (no error)=w495, Automation Refnum=refnum<k7> refnum ("Outlook._Application")) -> (Automation Refnum=w498:refnum<k7>, error out=w497:errorcluster)  [unwired: 2 in]
              n193 = invoke class="_Application" method="CreateItem"(reference=w498, error in=w497, "ItemType"=w491) -> (reference out=w492:refnum<k7>, error out=w493:errorcluster, "CreateItem"=w494:variant)  [unwired: 1 in, 1 out]
            }
          }
          n194 = Unbundle By Name(w459) -> ("Email"=w475:string, "S/N"=w473:string)
          n195 = Concatenate Strings("K5 - " ("string"), w473, " - Cosmed follow up" ("string")) -> (w471:string)
          n196 = Variant To Data(error in=w450, type=refnum<k7> refnum ("Outlook._MailItem"), Variant=w449) -> (data=w480:refnum<k7>, error out=w476:errorcluster)
          n197 = To Variant(anything=w464) -> (Variant=w467:variant)
          n198 = property class="_MailItem"(reference=w480, error in=w476, "To"=w475, "Subject"=w471) -> (reference out=w481:refnum<k7>, error out=w469:errorcluster, "Attachments"=w470:refnum<k7>)
          n199 = case shown="False" w461 {
            tunnel: w470 -> [w502 _]
            tunnel: w469 -> [w501 w503]
            tunnel: [w500 w503] -> w468
            tunnel: w467 -> [w499 _]
            frame False {
              n200 = invoke class="Attachments" method="Add"(reference=w502, error in=w501, "Source"=w499) -> (error out=w500:errorcluster)  [unwired: 4 in, 6 out]
            }
            frame True {
            }
          }
          n201 = invoke class="_MailItem" method="Display"(reference=w481, error in=w468) -> (reference out=w478:refnum<k7>, error out=w477:errorcluster)  [unwired: 2 in, 2 out]
          n202 = Close Reference(reference=w478, error in (no error)=w477) -> (error out=w482:errorcluster)
          n203 = Close Reference(reference=w451, error in (no error)=w482) -> (error out=w458:errorcluster)
        }
      }
    }
    frame Error {
    }
  }
  "error out" <- w3
  "reference out" <- w1
